vi "RealTimeChart.vi"() -> ()   [LabVIEW 2016, in "PCM MenuVIPanelSplit.lvclass"]
uses:
  PCM MenuVIPanelSplit.lvclass
  PanelSplitToolkit/PanelObject/PanelObject.lvclass
  Display Config.ctl
  Display Mode.ctl
  <vilib>/Analysis/4window.llb/windowTd.ctl
  <vilib>/Utility/miscctls.llb/LVRangeTypeDef.ctl
  PanelSplitToolkit/PanelDataNode/PanelDataNode.lvclass
  <vilib>/Utility/error.llb/DialogType.ctl
  PanelSplitToolkit/PanelDataNode/PanelDataNode.lvclass/PanelDataNode.ctl
  PanelSplitToolkit/PanelDataNode/Get RootQ.vi
  PanelSplitToolkit/QueueManager.llb/CreatQueue.vi
  PanelSplitToolkit/QueueManager.llb/Remove.vi
  PanelSplitToolkit/QueueManager.llb/Insert.vi
  PanelSplitToolkit/QueueManager.llb/Destroy.vi
  <vilib>/measure/NI_MABase.lvlib
  PCM PanelSplit.lvclass
  <vilib>/measure/NI_MAPro.lvlib
  <vilib>/Analysis/NI_AALPro.lvlib
  <vilib>/measure/maspectr.llb/FFT Power Spectrum and PSD for 1 Chan.vi
  <vilib>/measure/maspectr.llb/FFT Spectrum (Mag-Phase) for 1 Chan.vi
panel:
  out "Display":bool
  in  "Node*":refnum<data-value>
  out "波形图表":waveform(dbl)[](graph)
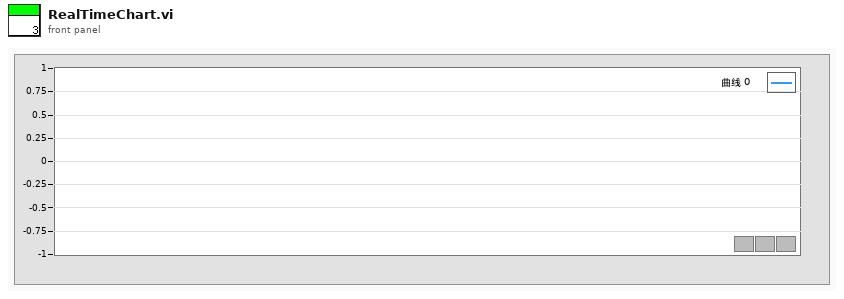
[diagram p1: front panel]
types:
  T1 = typedef "PCM PanelSplit.lvclass/Display Config.ctl" = cluster{"Display Mode":T2, "ChTag[]":string[], "window":T3, "Range":T4}
  T2 = typedef "PCM PanelSplit.lvclass/Display Mode.ctl" = enum16{"时域", "频谱", "功率谱"}
  T3 = typedef "NI_AALPro.lvlib/windowTd.ctl" = u32
  T4 = typedef "LVRangeTypeDef.ctl" = cluster{"Minimum":dbl, "Maximum":dbl, "Increment":dbl, "Minor Increment":dbl, "Start":dbl}
  T5 = cluster{"error":errorcluster, "LocalQ":cluster{"LQName":string, "LQEvent":string, "LQData":variant}, "HighQ":cluster{"HQName":string, "HQEvent":string, "HQData":variant}, "Display Config":T1, "波形图":refnum<vi>}
  T6 = typedef "DialogType.ctl" = u16
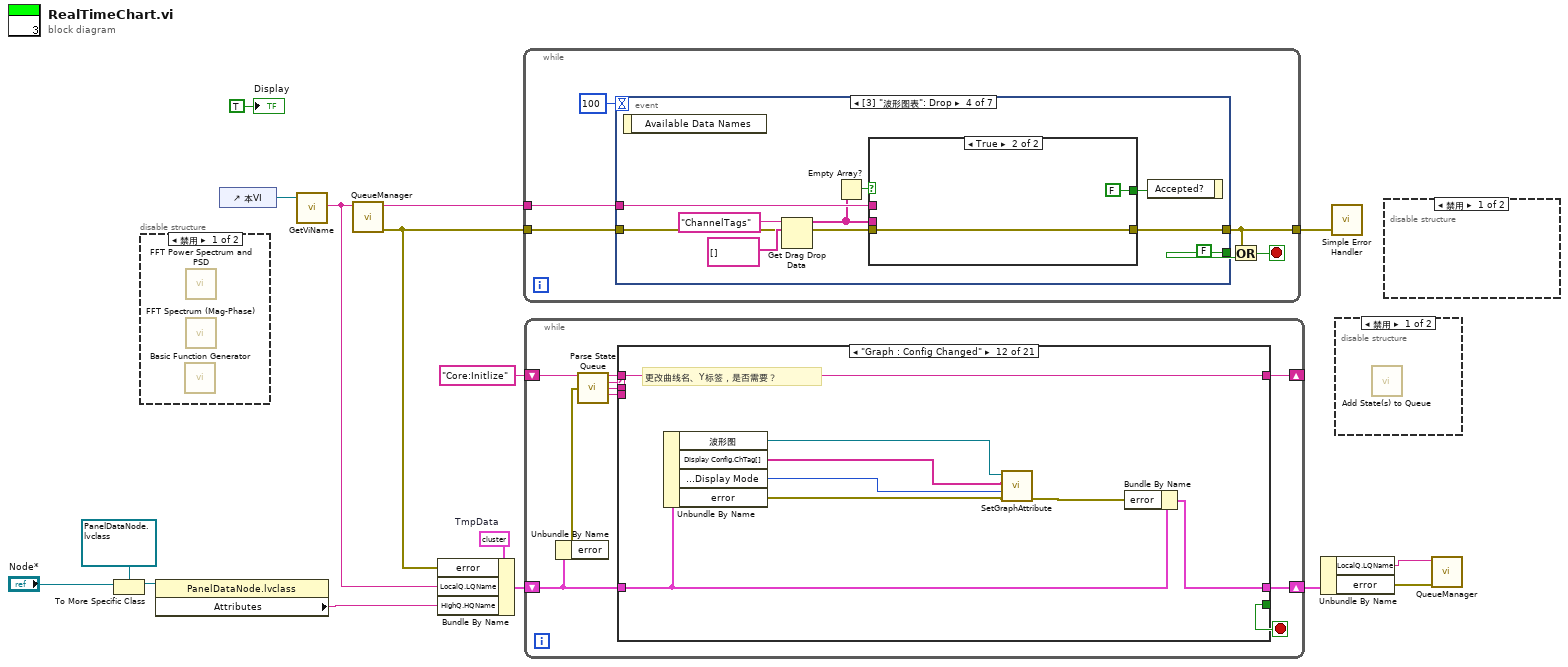
[diagram p0: block diagram]
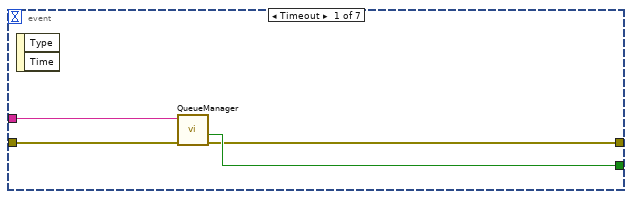
[diagram p5: hidden frame]
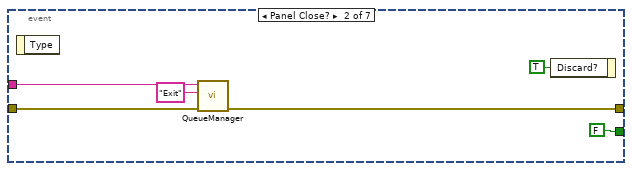
[diagram p6: hidden frame]
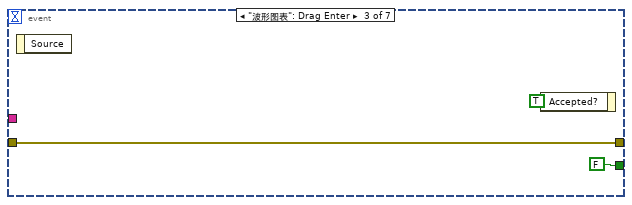
[diagram p7: hidden frame]
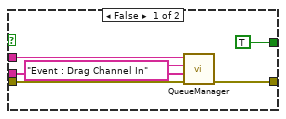
[diagram p8: hidden frame]
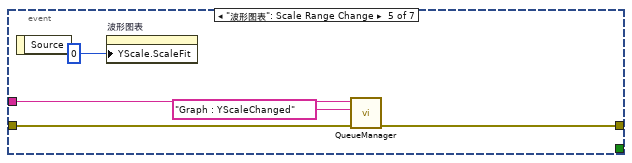
[diagram p9: hidden frame]
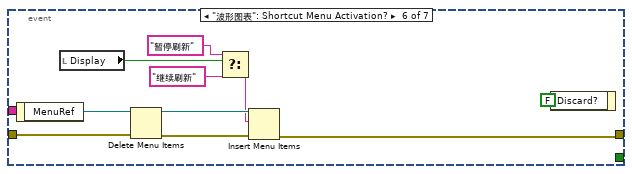
[diagram p10: hidden frame]
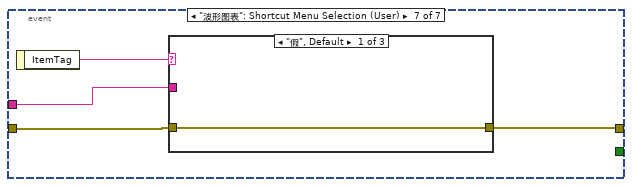
[diagram p11: hidden frame]
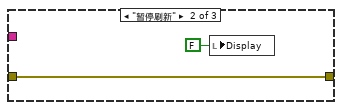
[diagram p12: hidden frame]
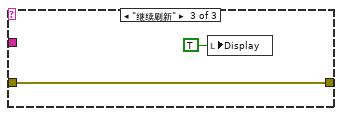
[diagram p13: hidden frame]
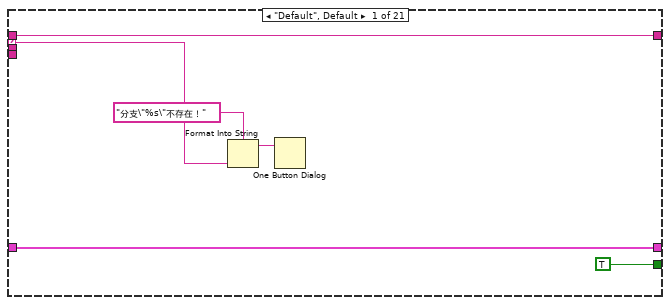
[diagram p14: hidden frame]
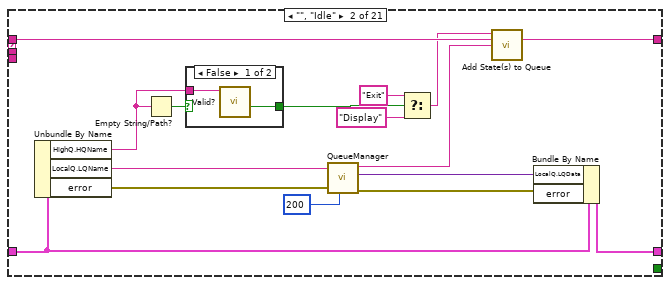
[diagram p15: hidden frame]
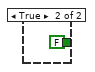
[diagram p16: hidden frame]
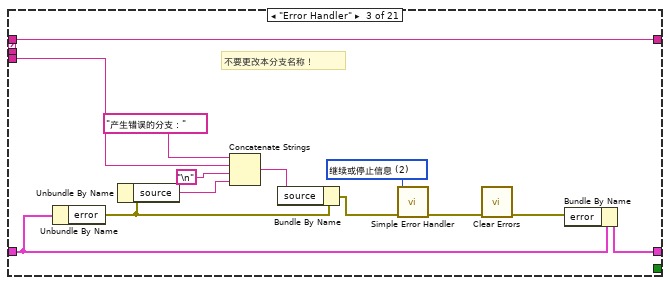
[diagram p17: hidden frame]
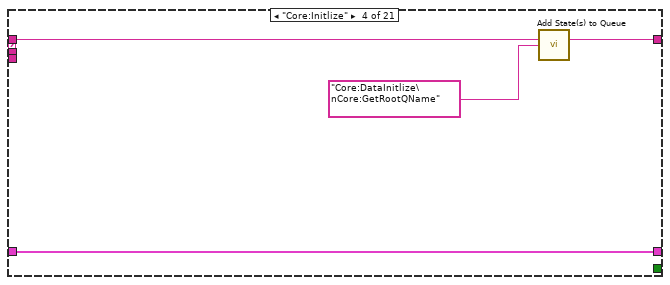
[diagram p18: hidden frame]
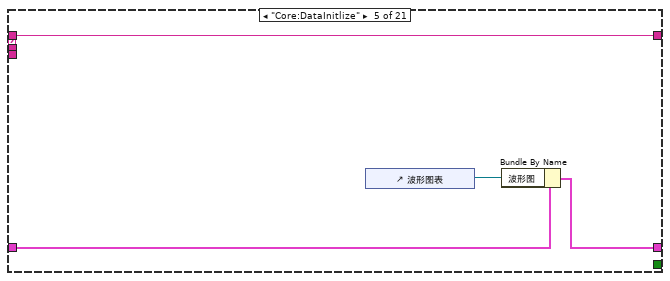
[diagram p19: hidden frame]
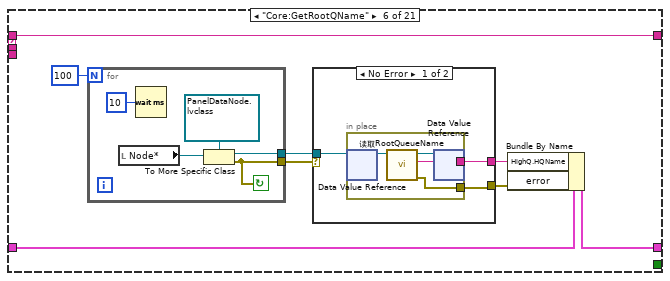
[diagram p20: hidden frame]
diagram:
  w12 = T5 {"error"={"status"=FALSE, "code"=0, "source"=""}, "LocalQ"={"LQName"="", "LQEvent"="", "LQData"=variant}, "HighQ"={"HQName"="", "HQEvent"="", "HQData"=variant}, "Display Config"={"Display Mode"=enum."时域", "ChTag[]"=[], "window"=0, "Range"={"Minimum"=0.0, "Maximum"=0.0, "Increment"=0.0, "Minor Increment"=0.0, "Start"=0.0}}, "波形图"=refnum}  # TmpData
  n1 = To More Specific Class(target class=refnum<data-value> refnum ("数据值引用"), reference="Node*") -> (specific class reference=w6:refnum<data-value>)  [unwired: 1 in, 1 out]
  n2 = disable-structure shown="禁用" {
    frame Disabled {
      n3 = call <vilib>:"Basic Function Generator.vi"() -> ()  [unwired: 9 in, 3 out]
      n4 = call-poly <vilib>:"FFT Power Spectrum and PSD.vi"() -> ()  [unwired: 8 in, 4 out]
      n5 = call-poly <vilib>:"FFT Spectrum (Mag-Phase).vi"() -> ()  [unwired: 7 in, 5 out]
    }
    frame Enabled {
    }
  }
  n6 = property class="PanelDataNode.lvclass"(reference=w6) -> ("Attributes"=w3:string)  [unwired: 1 in, 2 out]
  n7 = control-ref of="本VI"() -> (w7:refnum<vi>)
  n8 = call "GetViName.vi"("VI*"=w7) -> ("VI Name"=w8:string)  [unwired: 9 in, 1 out]
  n9 = call-poly "QueueManager.vi"("QueueName"=w8) -> ("error out"=w9:errorcluster, "QueueName out"=w1:string)  [unwired: 9 in]
  n10 = Bundle By Name(cluster=w12, "error"=w9, "LocalQ.LQName"=w8, "HighQ.HQName"=w3) -> (w11:T5)
  n11 = while {
    tunnel: w9 -> [w21]
    tunnel: w1 -> [w22]
    tunnel: [w18] -> w13
    stop <- w19 stop-if-true
    n12 = event shown="[3] \"波形图表\": Drop" {
      selector: _ -> [_ _ _ _ _ _ _]
      dyn-events: _ -> [_ _ _ _ _ _ _]
      timeout: 100 -> [_ _ _ _ _ _ _]
      tunnel: [w24 FALSE FALSE FALSE _ _ _] -> w20
      tunnel: w22 -> [w26 w31 _ w39 w54 _ w69]
      tunnel: w21 -> [w25 w30 w33 w41 w56 w60 w71]
      tunnel: [w23 w29 w33 w40 w55 w59 w68] -> w18
      event Timeout {
        n13 = event-data() -> ()  [unwired: 1 in, 2 out]
        n14 = call-poly "QueueManager.vi"("error in (no error)"=w25, "Queue Name(unamed)"=w26) -> ("error out"=w23:errorcluster, "Not Exist?"=w24:bool)  [unwired: 8 in]
      }
      event Panel Close? {
        n15 = event-data() -> ()  [unwired: 1 in, 1 out]
        n16 = call-poly "QueueManager.vi"("error in"=w30, "Event"="Exit", "QueueName"=w31) -> ("error out"=w29:errorcluster)  [unwired: 7 in, 1 out]
        n17 = event-data("Discard?"=TRUE ("放弃？")) -> ()  [unwired: 1 in, 1 out]
      }
      event "波形图表": Drag Enter {
        n18 = event-data() -> ()  [unwired: 1 in, 1 out]
        n19 = event-data("Accepted?"=TRUE ("放弃？")) -> ()  [unwired: 1 in, 1 out]
      }
      event "波形图表": Drop {
        n20 = event-data() -> ()  [unwired: 1 in, 1 out]
        n21 = Get Drag Drop Data(8:string[] [], 9:"ChannelTags" ("数据名称")) -> (3:w38:string[])  [unwired: 1 in, 1 out]
        n22 = Empty Array?(array=w38) -> (empty?=w37:bool)
        n23 = case shown="True" w37 {
          tunnel: w41 -> [w50 w52]
          tunnel: [w49 w52] -> w40
          tunnel: w39 -> [w48 _]
          tunnel: w38 -> [w46 _]
          tunnel: [TRUE ("放弃？") FALSE ("放弃？")] -> w36
          frame False {
            n24 = call-poly "QueueManager.vi"("error in"=w50, "Data"=w46, "Event"="Event : Drag Channel In", "QueueName"=w48) -> ("error out"=w49:errorcluster)  [unwired: 6 in, 1 out]
          }
          frame True {
          }
        }
        n25 = event-data("Accepted?"=w36) -> ()  [unwired: 1 in, 1 out]
      }
      event "波形图表": Scale Range Change {
        n26 = event-data() -> ()  [unwired: 1 in, 1 out]
        n27 = property on="波形图表" class="WFChart (strict)"("YScale.ScaleFit"=u8 0 ("Y标尺.标尺调节")) -> ()  [unwired: 2 in, 2 out]
        n28 = call-poly "QueueManager.vi"("error in"=w56, "Event"="Graph : YScaleChanged", "QueueName"=w54) -> ("error out"=w55:errorcluster)  [unwired: 7 in, 1 out]
      }
      event "波形图表": Shortcut Menu Activation? {
        n29 = event-data() -> ("MenuRef"=w67:refnum<k9>)  [unwired: 1 in]
        n30 = local read "Display"() -> (w64:bool)
        n31 = Delete Menu Items(6:w60, 9:w67) -> (0:w65:errorcluster, 3:w66:refnum<k9>)  [unwired: 2 in]
        n32 = Select(t="暂停刷新", s=w64, f="继续刷新") -> (s? t:f=w61:string)
        n33 = Insert Menu Items(6:w65, 8:w61, 9:w66) -> (0:w59:errorcluster)  [unwired: 3 in, 2 out]
        n34 = event-data("Discard?"=FALSE ("放弃？")) -> ()  [unwired: 1 in, 1 out]
      }
      event "波形图表": Shortcut Menu Selection (User) {
        n35 = event-data() -> ("ItemTag"=w70:string)  [unwired: 1 in]
        n36 = case shown="\"假\", Default" w70 {
          tunnel: w71 -> [w72 w74 w76]
          tunnel: w69 -> [_ _ _]
          tunnel: [w72 w74 w76] -> w68
          frame "假", Default {
          }
          frame "暂停刷新" {
            n37 = local write "Display"(FALSE ("Display")) -> ()
          }
          frame "继续刷新" {
            n38 = local write "Display"(TRUE ("Display")) -> ()
          }
        }
      }
    }
    n39 = Or(x=w18, y=w20) -> (x .or. y?=w19:bool)
  }
  n40 = while {
    shift-right: [w80] -> w14
    shift-left: w11 -> [w81]
    shift-right: [w79] -> _
    shift-left: "Core:Initlize" -> [w86]
    stop <- w83 stop-if-true
    n41 = Unbundle By Name(w81) -> ("error"=w82:errorcluster)
    n42 = call "Parse State Queue.vi"("State Queue"=w86, "Error In (no error)"=w82) -> ("Remaining States"=w85:string, "Current State"=w84:string, "Arguments"=w78:string, "PreState"=w77:string)  [unwired: 10 in]
    n43 = case shown="\"Graph : Config Changed\"" w84 {
      selector: w84 -> [w90 _ _ _ _ _ _ _ _ _ _ _ _ _ _ _ _ _ _ _ _]
      tunnel: w85 -> [w91 w105 w124 w127 w132 w140 _ _ w161 w169 w182 w204 w210 w212 w216 w231 w243 w255 w265 w280 w281]
      tunnel: w78 -> [_ _ _ _ _ _ _ _ _ _ _ _ _ _ _ _ _ _ _ _ _]
      tunnel: [TRUE _ _ _ _ _ TRUE FALSE FALSE _ _ _ _ _ _ _ _ _ _ _ _] -> w83
      tunnel: w81 -> [w92 w102 w121 w128 w131 w136 w156 w159 w162 w171 w179 w200 w211 w213 w220 w233 w245 w259 w269 w275 w282]
      tunnel: [w92 w107 w120 w128 w130 w135 w156 w159 w162 w170 w177 w198 w207 w213 w219 w232 w244 w258 w268 w273 w282] -> w80
      tunnel: [w91 w104 w124 w126 w132 w140 "" ("Remaining States") "Core:Exit" ("Remaining States") w161 w168 w182 w204 w209 w212 w215 w230 w242 w254 w264 w280 w281] -> w79
      tunnel: w77 -> [_ _ w118 _ _ _ _ _ _ _ _ _ _ _ _ _ _ _ _ _ _]
      frame "Default", Default {
        n44 = Format Into String(format string="分支\"%s\"不存在！" ("格式字符串"), w90) -> (resulting string=w89:string)  [unwired: 2 in, 1 out]
        n45 = One Button Dialog(message=w89) -> ()  [unwired: 1 in, 1 out]
      }
      frame "", "Idle" {
        n46 = Unbundle By Name(w102) -> ("HighQ.HQName"=w96:string, "LocalQ.LQName"=w101:string, "error"=w100:errorcluster)
        n47 = Empty String/Path?(string/path=w96) -> (empty?=w99:bool)
        n48 = case shown="False" w99 {
          tunnel: [w110 FALSE ("Not Exist?")] -> w98
          tunnel: w96 -> [w109 _]
          frame False {
            n49 = call "Valid?.vi"("Queue Name(unamed)"=w109) -> ("Not Exist?"=w110:bool)  [unwired: 9 in, 1 out]
          }
          frame True {
          }
        }
        n50 = call-poly "QueueManager.vi"("Time out(-1)"=200, "error in (no error)"=w100, "Queue Name"=w101) -> ("error out"=w108:errorcluster, "Data"=w106:variant, "Event"=w95:string)  [unwired: 5 in, 1 out]
        n51 = Select(t="Exit" ("Event"), s=w98, f="Display") -> (s? t:f=w94:string)
        n52 = call "Add State(s) to Queue.vi"("State(s) in Front (\"\")"=w94, "State(s) in (\"\")"=w105, "State(s) at Back (\"\")"=w95) -> ("States Out"=w104:string)  [unwired: 12 in]
        n53 = Bundle By Name(cluster=w102, "LocalQ.LQData"=w106, "error"=w108) -> (w107:T5)
      }
      frame "Error Handler" {
        w119 = T6 2 items=["无对话框", "确定信息", "继续或停止信息", "确定信息＋警告", "继续/停止+警告"] ("type of dialog (OK msg:1)")
        # "不要更改本分支名称！"
        n54 = Unbundle By Name(w121) -> ("error"=w113:errorcluster)
        n55 = Unbundle By Name(w113) -> ("source"=w116:string)
        n56 = Concatenate Strings("产生错误的分支：" ("字符串"), w118, "\n", w116) -> (w114:string)
        n57 = Bundle By Name(cluster=w113, "source"=w114) -> (w112:errorcluster)
        n58 = call <vilib>:"Simple Error Handler.vi"("type of dialog (OK msg:1)"=w119, "error in (no error)"=w112) -> ("error out"=w122:errorcluster)  [unwired: 3 in, 4 out]
        n59 = call <vilib>:"Clear Errors.vi"("error in (no error)"=w122) -> ("error out"=w123:errorcluster)  [unwired: 5 in, 1 out]
        n60 = Bundle By Name(cluster=w121, "error"=w123) -> (w120:T5)
      }
      frame "Core:Initlize" {
        n61 = call "Add State(s) to Queue.vi"("State(s) in (\"\")"=w127, "State(s) at Back (\"\")"="Core:DataInitlize\nCore:GetRootQName" ("State(s) at Back (\"\")")) -> ("States Out"=w126:string)  [unwired: 13 in]
      }
      frame "Core:DataInitlize" {
        n62 = control-ref of="波形图表"() -> (w129:refnum<vi>)
        n63 = Bundle By Name(cluster=w131, "波形图"=w129) -> (w130:T5)
      }
      frame "Core:GetRootQName" {
        n64 = for {
          N: 100 -> [_]
          tunnel: [w152] -> w137
          tunnel: [w151] -> w134
          stop <- w151 continue-if-true
          n65 = local read "Node*"() -> (w154:refnum<data-value>)
          n66 = Wait (ms)(milliseconds to wait=u32 10 ("等待时间（毫秒）")) -> ()  [unwired: 1 out]
          n67 = To More Specific Class(target class=refnum<data-value> refnum ("Node*"), reference=w154) -> (specific class reference=w152:refnum<data-value>, error out=w151:errorcluster)  [unwired: 1 in]
        }
        n68 = case shown="No Error" w134 {
          selector: w134 -> [_ w149]
          tunnel: [w141 w149] -> w139
          tunnel: [w143 "" ("RootQueueName")] -> w138
          tunnel: w137 -> [w142 _]
          frame No Error {
            n69 = in-place {
              in-place-border: [w145] -> w143
              in-place-border: [w144] -> w141
              n70 = in-place-dvr #1(w142) -> (w147:refnum<class "PanelDataNode.lvclass">)  [unwired: 1 out]
              n71 = call "读取RootQueueName.vi"("PanelDataNode输入"=w147) -> ("error out"=w144:errorcluster, "RootQueueName"=w145:string, "PanelDataNode输出"=w146:refnum<class "PanelDataNode.lvclass">)  [unwired: 8 in]
              n72 = in-place-dvr #1(w146) -> ()  [unwired: 2 out]
            }
          }
          frame Error {
          }
        }
        n73 = Bundle By Name(cluster=w136, "HighQ.HQName"=w138, "error"=w139) -> (w135:T5)
      }
      frame "Core:Exit" {
      }
      frame "Exit" {
      }
      frame "-----User Event------" {
      }
      frame "Event : Drag Channel In" {
        # "可考虑做成增加通道而不是替换通道的效果，但是需要有机制能删除通道，暂时用替换模式。"
        n74 = Unbundle By Name(w171) -> ("Display Config.ChTag[]"=w173:string[], "LocalQ.LQData"=w174:variant, "error"=w175:errorcluster)
        n75 = property on="波形图表" class="WFChart (strict)"("YScale.ScaleFit"=u8 2 ("Y标尺.标尺调节")) -> ()  [unwired: 2 in, 2 out]
        n76 = Variant To Data(error in=w175, type=w173, Variant=w174) -> (data=w166:string[], error out=w172:errorcluster)
        n77 = Bundle By Name(cluster=w171, "HighQ.HQEvent"="Rec : Source Changed", "HighQ.HQData"=w166, "Display Config.ChTag[]"=w166, "error"=w172) -> (w170:T5)
        n78 = call "Add State(s) to Queue.vi"("State(s) in Front (\"\")"="Com : Send To RootPanel\nGraph : Config Changed", "State(s) in (\"\")"=w169) -> ("States Out"=w168:string)  [unwired: 13 in]
      }
      frame "Display" {
        n79 = Unbundle By Name(w179) -> ("Display Config"=w181:T1, "error"=w180:errorcluster)
        n80 = Wait (ms)(milliseconds to wait=u32 50 ("等待时间（毫秒）")) -> ()  [unwired: 1 out]
        n81 = disable-structure shown="启用" {
          disable-tunnel: w181 -> [w187 w195]
          disable-tunnel: w180 -> [w186 w191]
          disable-tunnel: [w183 w190] -> w178
          frame Disabled {
            n82 = call "GetDisplayData.vi"("error in"=w186, "Display Config"=w187) -> ("error out"=w183:errorcluster, "Data"=w185:cluster{"f0":dbl, "df":dbl, "magnitude":dbl[]}[], "Valid?"=w184:bool)  [unwired: 7 in]
            n83 = case shown="True" w184 {
              tunnel: w185 -> [_ _]
              frame False {
              }
              frame True {
              }
            }
          }
          frame Enabled {
            n84 = Unbundle By Name(w195) -> ("ChTag[]"=w192:string[])
            n85 = local read "Display"() -> (w194:bool)
            n86 = call "Api_GetWaveform.vi"("error in (no error)"=w191, "Tags[]"=w192) -> ("error out"=w190:errorcluster, "Display?"=w188:bool, "Wave[]"=w189:waveform(dbl)[])  [unwired: 7 in]
            n87 = And(x=w194, y=w188) -> (x .and. y?=w193:bool)
            n88 = case shown="True" w193 {
              tunnel: w189 -> [_ w196]
              frame False {
              }
              frame True {
                "波形图表" <- w196
              }
            }
          }
        }
        n89 = Bundle By Name(cluster=w179, "error"=w178) -> (w177:T5)
      }
      frame "Graph : Config Changed" {
        # "更改曲线名、Y标签，是否需要？"
        n90 = Unbundle By Name(w200) -> ("波形图"=w203:refnum<vi>, "Display Config.ChTag[]"=w197:string[], "Display Config.Display Mode"=w202:T2, "error"=w201:errorcluster)
        n91 = call "SetGraphAttribute.vi"("error in"=w201, "Display Mode"=w202, "CH Tag[]"=w197, "波形图表"=w203) -> ("error out"=w199:errorcluster)  [unwired: 7 in]
        n92 = Bundle By Name(cluster=w200, "error"=w199) -> (w198:T5)
      }
      frame "Graph : YScaleChanged" {
        # "Com : Send To RootPanel"
        n93 = property on="波形图表" class="WFChart (strict)"() -> ("YScale.Range"=w205:T4)  [unwired: 2 in, 2 out]
        n94 = Bundle By Name(cluster=w211, "HighQ.HQEvent"="Rec : YScaleChanged", "HighQ.HQData"=w205) -> (w207:T5)
        n95 = call "Add State(s) to Queue.vi"("State(s) in Front (\"\")"="Com : Send To RootPanel" ("State(s) in Front (\"\")"), "State(s) in (\"\")"=w210) -> ("States Out"=w209:string)  [unwired: 13 in]
      }
      frame "---Communication---" {
      }
      frame "Rec : Channel Changed" {
        n96 = Unbundle By Name(w220) -> ("Display Config.ChTag[]"=w221:string[], "LocalQ.LQData"=w222:variant, "error"=w223:errorcluster)
        n97 = Variant To Data(error in=w223, type=w221, Variant=w222) -> (data=w217:string[], error out=w218:errorcluster)
        n98 = Bundle By Name(cluster=w220, "Display Config.ChTag[]"=w217, "error"=w218) -> (w219:T5)
        n99 = call "Add State(s) to Queue.vi"("State(s) in Front (\"\")"="Graph : Config Changed", "State(s) in (\"\")"=w216) -> ("States Out"=w215:string)  [unwired: 13 in]
      }
      frame "Rec : UpdataConfig" {
        # "需要考虑通道名称改变、勾选改变等情况"
        # "配置信息进行了更改"
        n100 = Unbundle By Name(w233) -> ("Display Config.ChTag[]"=w228:string[], "error"=w229:errorcluster)
        n101 = Empty Array?(array=w228) -> (empty?=w227:bool)
        n102 = Select(t="", s=w227, f="Graph : Config Changed") -> (s? t:f=w224:string)
        n103 = call "Add State(s) to Queue.vi"("State(s) in Front (\"\")"=w224, "State(s) in (\"\")"=w231) -> ("States Out"=w230:string)  [unwired: 13 in]
        n104 = Bundle By Name(cluster=w233, "error"=w229) -> (w232:T5)
      }
      frame "Rec : Load" {
        n105 = Unbundle By Name(w245) -> ("LocalQ.LQData"=w246:variant, "error"=w247:errorcluster)
        n106 = Variant To Data(error in=w247, type=T1 {"Display Mode"=enum."时域", "ChTag[]"=[], "window"=1, "Range"={"Minimum"=0.0, "Maximum"=0.0, "Increment"=0.0, "Minor Increment"=0.0, "Start"=0.0}} ("Display Config"), Variant=w246) -> (data=w238:T1, error out=w241:errorcluster)
        n107 = Unbundle By Name(w238) -> ("Range"=w236:T4)
        n108 = Equal?(x=w236, y=T4 {"Minimum"=0.0, "Maximum"=0.0, "Increment"=0.0, "Minor Increment"=0.0, "Start"=0.0} ("Range")) -> (x = y?=w234:bool)
        n109 = case shown="False" w234 {
          tunnel: w241 -> [w251 w252]
          tunnel: [w250 w252] -> w240
          tunnel: w236 -> [w248 _]
          frame False {
            n110 = property on="波形图表" class="WFChart (strict)"(error in=w251, "YScale.ScaleFit"=u8 0 ("Y标尺.标尺调节"), "YScale.Range"=w248) -> (error out=w250:errorcluster)  [unwired: 1 in, 1 out]
          }
          frame True {
          }
        }
        n111 = Bundle By Name(cluster=w245, "Display Config"=w238, "error"=w240) -> (w244:T5)
        n112 = call "Add State(s) to Queue.vi"("State(s) in Front (\"\")"="Graph : Config Changed", "State(s) in (\"\")"=w243) -> ("States Out"=w242:string)  [unwired: 13 in]
      }
      frame "Rec : Window Changed" {
        n113 = Unbundle By Name(w259) -> ("Display Config.window"=w260:T3, "LocalQ.LQData"=w261:variant, "error"=w262:errorcluster)
        n114 = Variant To Data(error in=w262, type=w260, Variant=w261) -> (data=w256:T3, error out=w257:errorcluster)
        n115 = Bundle By Name(cluster=w259, "Display Config.window"=w256, "error"=w257) -> (w258:T5)
        n116 = call "Add State(s) to Queue.vi"("State(s) in Front (\"\")"="Graph : Config Changed", "State(s) in (\"\")"=w255) -> ("States Out"=w254:string)  [unwired: 13 in]
      }
      frame "Rec : DisplayMode Changed" {
        n117 = Unbundle By Name(w269) -> ("Display Config.Display Mode"=w270:T2, "LocalQ.LQData"=w271:variant, "error"=w272:errorcluster)
        n118 = Variant To Data(error in=w272, type=w270, Variant=w271) -> (data=w266:T2, error out=w267:errorcluster)
        n119 = Bundle By Name(cluster=w269, "Display Config.Display Mode"=w266, "error"=w267) -> (w268:T5)
        n120 = call "Add State(s) to Queue.vi"("State(s) in (\"\")"=w265, "State(s) at Back (\"\")"="Graph : Config Changed") -> ("States Out"=w264:string)  [unwired: 13 in]
      }
      frame "Com : Send To RootPanel" {
        n121 = Unbundle By Name(w275) -> ("HighQ.HQName"=w276:string, "HighQ.HQEvent"=w277:string, "HighQ.HQData"=w278:variant, "error"=w279:errorcluster)
        n122 = call-poly "QueueManager.vi"("error in"=w279, "Data"=w278, "Event"=w277, "QueueName"=w276) -> ("error out"=w274:errorcluster)  [unwired: 6 in, 1 out]
        n123 = Bundle By Name(cluster=w275, "error"=w274) -> (w273:T5)
      }
      frame "Send : Channel Changed" {
      }
    }
  }
  n124 = Unbundle By Name(w14) -> ("LocalQ.LQName"=w10:string, "error"=w15:errorcluster)
  n125 = call <vilib>:"Simple Error Handler.vi"("error in (no error)"=w13) -> ()  [unwired: 4 in, 5 out]
  n126 = disable-structure shown="禁用" {
    frame Disabled {
      n127 = call "Add State(s) to Queue.vi"() -> ()  [unwired: 15 in, 1 out]
    }
    frame Enabled {
    }
  }
  n128 = disable-structure shown="禁用" {
    frame Disabled {
    }
    frame Enabled {
    }
  }
  n129 = call-poly "QueueManager.vi"("error in (no error)"=w15, "QueeuName"=w10) -> ()  [unwired: 9 in, 1 out]
  "Display" <- TRUE ("PauseDisplay")
